vi "Update Group.vi"(6 "dt":dbl, 8 "error in (no error)":errorcluster, 9 "t0":dbl, 10 "Data":dbl[][](array[numeric]), 11 "DataProcessor in":refnum<class "DataProcessor.lvclass">) -> (0 "error out":errorcluster, 3 "DataProcessor out":refnum<class "DataProcessor.lvclass">)   [LabVIEW 2020, in "Volatus.lvlib" / "DataProcessor.lvclass"]
uses:
  DataProcessor.lvclass
  C:/dev/lv20CE/relink/lv-volatus/Volatus/Task/Task.lvclass
  DataProcessor.lvclass/DataProcessor.ctl
  Task/Task.lvclass/Task.ctl
  TelemetryAPI/TelemetryAPI.lvclass/TelemetryAPI.ctl
  lv-vecto/Vecto/Group/Group.lvclass
  C:/dev/lv20CE/relink/lv-vecto/Vecto/GroupAbstract/GroupAbstract.lvclass
  <vilib>/Analysis/baseanly.llb/Mean (DBL).vi
  <vilib>/Analysis/NI_AALBase.lvlib
  Task/Task.lvclass
  C:/dev/lv20CE/relink/lv-vecto/Vecto/Group/Group.lvclass
  C:/dev/lv20CE/relink/lv-volatus/Volatus/DataHandlerTask/DataHandlerTask.lvclass
  C:/Program Files (x86)/National Instruments/LabVIEW 2020/vi.lib/ActorFramework/Actor/Actor.lvclass
  C:/dev/lv20CE/relink/lv-volatus/Volatus/TaskStateHandler/TaskStateHandler.lvclass
  C:/dev/lv20CE/relink/lv-volatus/Volatus/VectoMessageHandler/VectoMessageHandler.lvclass
  C:/dev/lv20CE/relink/lv-volatus/Volatus/API Provider/API Provider.lvclass
  C:/dev/lv20CE/relink/lv-volatus/Volatus/DataHandler/DataHandler.lvclass
  C:/dev/lv20CE/relink/lv-volatus/Volatus/DataProcessor/DataProcessor.lvclass
  C:/dev/lv20CE/relink/lv-volatus/Volatus/Abortable/Abortable.lvclass
  C:/dev/lv20CE/relink/lv-volatus/Volatus/Reconfigurable/Reconfigurable.lvclass
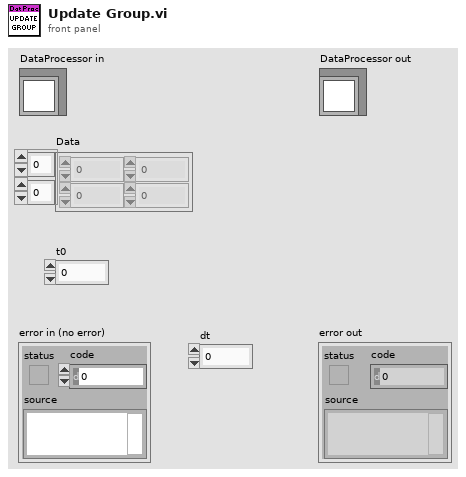
[diagram p1: front panel]
types:
  T1 = typedef "Volatus.lvlib/Decimation Type.ctl" = enum16{"Mean", "Latest"}
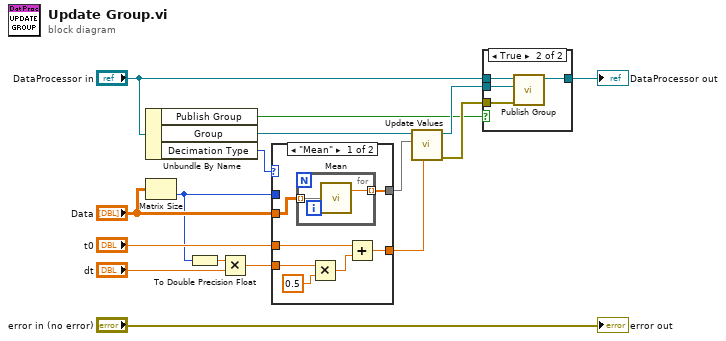
[diagram p0: block diagram]
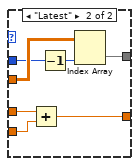
[diagram p3: hidden frame]
diagram:
  n1 = Unbundle By Name("DataProcessor in") -> ("Publish Group"=w1:bool, "Group"=w7:refnum<class "Group.lvclass">, "Decimation Type"=w14:T1)
  n2 = Matrix Size(0:"Data") -> (2:w8:i32)  [unwired: 1 out]
  n3 = To Double Precision Float(number=w8) -> (double precision float=w12:dbl)
  n4 = Multiply(x=w12, y="dt") -> (x*y=w11:dbl)
  n5 = case shown="\"Mean\"" w14 {
    tunnel: w11 -> [w23 w31]
    tunnel: "t0" -> [w21 w32]
    tunnel: "Data" -> [w18 w29]
    tunnel: [w19 w30] -> w5
    tunnel: w8 -> [_ w28]
    tunnel: [w17 w26] -> w6
    frame "Mean" {
      n6 = for {
        tunnel: w18 -> [w25] mode=indexing
        tunnel: [w24] -> w17 mode=indexing
        n7 = call-poly <vilib>:"Mean.vi"("X"=w25) -> ("mean"=w24:dbl)  [unwired: 1 out]
      }
      n8 = Multiply(x=w23, y=0.5) -> (x*y=w20:dbl)
      n9 = Add(x=w21, y=w20) -> (x+y=w19:dbl)
    }
    frame "Latest" {
      n10 = Add(x=w32, y=w31) -> (x+y=w30:dbl)
      n11 = Decrement(x=w28) -> (x-1=w27:i32)
      n12 = Index Array(array=w29, index (col)=w27) -> (element=w26:dbl[])  [unwired: 1 in]
    }
  }
  n13 = call "Update Values.vi"("Timestamp (Now)"=w5, "Values"=w6, "Group in"=w7) -> ("error out"=w2:errorcluster, "Group out"=w3:refnum<class "Group.lvclass">)  [unwired: 7 in]
  n14 = case shown="True" w1 {
    tunnel: "DataProcessor in" -> [w33 w37]
    tunnel: [w33 w36] -> w4
    tunnel: w3 -> [_ w35]
    tunnel: w2 -> [_ w34]
    frame False {
    }
    frame True {
      n15 = call "Publish Group.vi"("error in (no error)"=w34, "Group"=w35, "Task in"=w37) -> ("Task out"=w36:refnum<class "DataProcessor.lvclass">)  [unwired: 7 in, 1 out]
    }
  }
  "DataProcessor out" <- w4
  "error out" <- "error in (no error)"
